vi "CSM-LogViewer(WhileLoop).vi"() -> ()   [LabVIEW 2020]
uses:
  <userlib>/_NEVSTOP/Communicable State Machine(CSM)/_Support/Common/Trim Single line Text.vi
  <userlib>/_NEVSTOP/Communicable State Machine(CSM)/_Support/Common/Format Timestamp.vi
  <userlib>/_NEVSTOP/Communicable State Machine(CSM)/Communicable State Machine.lvlib
panel:
  in  "read line":bool
  in  "stop":bool
  in  "Array":cluster{"CSM":string, "Message":string}[](array[cluster])=[{"CSM"="DH1766", "Message"="MeasureAllVC(Complete)"}, {"CSM"="DH1766", "Message"="MeasureAllVC"}, {"CSM"="IT6900-2", "Message"="MeasureAllVC"}, {"CSM"="IT6900-2", "Message"="MeasureAllVC(Complete)"}, {"CSM"="电流监控", "Message"="Action: Check Current"}, {"CSM"="电流监控", "Message"="Action: Update Status"}, {"CSM"="电流监控", "Message"="Action: Continous Check"}, {"CSM"="电流监控", "Message"="Action: Continous Check(Complete)"}, {"CSM"="YX10A", "Message"="Action: Send R2 and R4"}, {"CSM"="YX10A", "Message"="Action: Continue Check"}, {"CSM"="YX10A", "Message"="Action: Continue Check(Complete)"}]
  out "String Cache":string="[11:08:49.216] [2024/7/18 12:18:43]  [Module Destroyed] CSM-Script-Window\r\n\r[11:08:49.214] [2024/7/18 12:18:43]  [State Change] CSM-Script-Window | <Remaining States> >> <Empty>\r\n\r[11:08:49.212] [2024/7/18 12:18:43]  [State Change] CSM-Script-Window | Exit\r\n\r[11:08:49.210] [2024/7/18 12:18:43]  [State Change] CSM-Script-Window | Events: Unregister\r\n\r[11:08:49.207] [2024/7/18 12:18:43]  [State Change] CSM-Script-Window | Data: Cleanup\r\n\r[11:08:49.205] [2024/7/18 12:18:43]  [State Change] CSM-Script-Window | Macro: Exit(Complete) <- -SendMsgAPI95F21AFF29B0\r\n\r[11:08:49.203] [2024/7/18 12:18:43]  [State Change] CSM-Script-Window | Macro: Exit <- -SendMsgAPI95F21AFF29B0\r\n\r[11:08:49.200] [2024/7/18 12:17:39]  [State Change] CSM-Script-Window | \r\n\r[11:08:49.199] [2024/7/18 12:17:39]  [State Change] Switch2737 | Close(Complete) <- CSM-Script-Window\r\n\r[11:08:49.196] [2024/7/18 12:17:39]  [State Change] Switch2737 | Close <- CSM-Script-Window\r\n\r[11:08:49.194] [2024/7/18 12:17:39]  [User Log] CMD | Close -@ Switch2737\r\n\r[11:08:49.192] [2024/7/18 12:17:39]  [State Change] NI6349DO | Close(Complete) <- CSM-Script-Window\r\n\r[11:08:49.190] [2024/7/18 12:17:39]  [User Log] NI6349DO | Close >> {reset:TRUE}\r\n\r[11:08:49.188] [2024/7/18 12:17:39]  [State Change] NI6349DO | Close <- CSM-Script-Window\r\n\r[11:08:49.186] [2024/7/18 12:17:39]  [User Log] CMD | Close -@ NI6349DO\r\n\r[11:08:49.184] [2024/7/18 12:17:39]  [State Change] NI6509DO | Close(Complete) <- CSM-Script-Window\r\n\r[11:08:49.182] [2024/7/18 12:17:39]  [User Log] NI6509DO | Close >> {reset:TRUE}\r\n\r[11:08:49.180] [2024/7/18 12:17:39]  [State Change] NI6509DO | Close <- CSM-Script-Window\r\n\r[11:08:49.178] [2024/7/18 12:17:39]  [User Log] CMD | Close -@ NI6509DO\r\n\r[11:08:49.176] [2024/7/18 12:17:39]  [State Change] NI6349AI | Close(Complete) <- CSM-Script-Window\r\n\r[11:08:49.174] [2024/7/18 12:17:39]  [State Change] NI6349AI | Close <- CSM-Script-Window\r\n\r[11:08:49.172] [2024/7/18 12:17:39]  [User Log] CMD | Close -@ NI6349AI\r\n\r[11:08:49.170] [2024/7/18 12:17:39]  [State Change] DL850E | Close(Complete) <- CSM-Script-Window\r\n\r[11:08:49.168] [2024/7/18 12:17:39]  [State Change] DL850E | Close <- CSM-Script-Window\r\n\r[11:08:49.166] [2024/7/18 12:17:39]  [User Log] CMD | Close -@ DL850E\r\n\r[11:08:49.164] [2024/7/18 12:17:39]  [State Change] TargetSim | Close(Complete) <- CSM-Script-Window\r\n\r[11:08:49.161] [2024/7/18 12:17:39]  [State Change] TargetSim | Close <- CSM-Script-Window\r\n\r[11:08:49.159] [2024/7/18 12:17:39]  [User Log] CMD | Close -@ TargetSim\r\n\r[11:08:49.157] [2024/7/18 12:17:39]  [State Change] TM10A | Close(Complete) <- CSM-Script-Window\r\n\r[11:08:49.155] [2024/7/18 12:17:39]  [State Change] TM10A | Close <- CSM-Script-Window\r\n\r[11:08:49.153] [2024/7/18 12:17:39]  [User Log] CMD | Close -@ TM10A\r\n\r[11:08:49.151] [2024/7/18 12:17:39]  [State Change] Safe10A | Close(Complete) <- CSM-Script-Window\r\n\r[11:08:49.149] [2024/7/18 12:17:38]  [State Change] Safe10A | Close <- CSM-Script-Window\r\n\r[11:08:49.147] [2024/7/18 12:17:38]  [User Log] CMD | Close -@ Safe10A\r\n\r[11:08:49.145] [2024/7/18 12:17:38]  [State Change] YX10A | Action: Stop Sending R2 and R4(Complete) <- <end>\r\n\r[11:08:49.143] [2024/7/18 12:17:38]  [State Change] YX10A | Action: Stop Sending R2 and R4 <- <end>\r\n\r[11:08:49.141] [2024/7/18 12:17:38]  [State Change] YX10A | Close(Complete) <- CSM-Script-Window\r\n\r[11:08:49.139] [2024/7/18 12:17:38]  [State Change] YX10A | Close <- CSM-Script-Window\r\n\r[11:08:49.137] [2024/7/18 12:17:38]  [User Log] CMD | Close -@ YX10A\r\n\r[11:08:49.135] [2024/7/18 12:17:38]  [State Change] DH1766 | Close(Complete) <- CSM-Script-Window\r\n\r[11:08:48.357] [2024/7/18 12:17:37]  [State Change] DH1766 | Close <- CSM-Script-Window\r\n\r[11:08:48.355] [2024/7/18 12:17:37]  [User Log] CMD | Close -@ DH1766\r\n\r[11:08:48.353] [2024/7/18 12:17:37]  [State Change] DH1766 | Output(Complete) >> FALSE;2 <- CSM-Script-Window\r\n\r[11:08:48.298] [2024/7/18 12:17:37]  [Error Log] Safe10A | Error: -1073807298 >> [Error: -1073807298]VISA Read in Safe.lvlib:Safe(10A).vi%2D%3E10A - COMCSMs.vi%2D%3E10A - CSMs(Without DCPower).vi%2D%3E10A - CSMs.vi\r\n\r[11:08:48.021] [2024/7/18 12:17:37]  [State Change] DH1766 | Output >> FALSE;2 <- CSM-Script-Window\r\n\r[11:08:48.017] [2024/7/18 12:17:37]  [User Log] CMD | Output >> FALSE;2 -@ DH1766\r\n\r[11:08:48.006] [2024/7/18 12:17:36]  [State Change] IT6900-2 | Close(Complete) <- CSM-Script-Window\r\n\r[11:08:47.996] [2024/7/18 12:17:36]  [State Change] IT6900-2 | Close <- CSM-Script-Window\r\n\r[11:08:47.989] [2024/7/18 12:17:36]  [User Log] CMD | Close -@ IT6900-2\r\n\r[11:08:47.988] [2024/7/18 12:17:36]  [State Change] IT6900-2 | Output(Complete) >> FALSE;0 <- CSM-Script-Window\r\n\r[11:08:47.985] [2024/7/18 12:17:36]  [State Change] IT6900-2 | Output >> FALSE;0 <- CSM-Script-Window\r\n\r[11:08:47.983] [2024/7/18 12:17:36]  [User Log] CMD | Output >> FALSE;0 -@ IT6900-2\r\n\r[11:08:47.982] [2024/7/18 12:17:36]  [State Change] 电流监控 | UI: Front Panel State(Complete) >> Close <- CSM-Script-Window\r\n\r[11:08:47.974] [2024/7/18 12:17:36]  [State Change] 电流监控 | UI: Front Panel State >> Close <- CSM-Script-Window\r\n\r[11:08:47.972] [2024/7/18 12:17:36]  [State Change] 电流监控 | Action: Update Status(Complete) <- <end>\r\n\r[11:08:47.965] [2024/7/18 12:17:36]  [User Log] CMD | UI: Front Panel State >> Close -@ 电流监控\r\n\r[11:08:47.961] [2024/7/18 12:17:36]  [State Change] 电流监控 | Action: Finish Monitoring\r\n\r[11:08:47.957] [2024/7/18 12:17:36]  [State Change] 电流监控 | 停止电流监控(Complete) <- CSM-Script-Window\r\n\r[11:08:47.955] [2024/7/18 12:17:36]  [State Change] 电流监控 | 停止电流监控 <- CSM-Script-Window\r\n\r[11:08:47.922] [2024/7/18 12:17:36]  [User Log] CMD | 停止电流监控 -@ 电流监控\r\n\r[11:08:47.908] [2024/7/18 12:17:36]  [State Change] DUTCTRL | ALOG_R(Complete) >> FALSE <- CSM-Script-Window\r\n\r[11:08:47.906] [2024/7/18 12:17:36]  [State Change] NI6509DO | WriteLine(Complete) >> {Line:PXIe-6509/port1/line1;Value:FALSE} <- -SendMsgAPIBD11725CA234\r\n\r[11:08:47.903] [2024/7/18 12:17:36]  [State Change] NI6509DO | WriteLine >> {Line:PXIe-6509/port1/line1;Value:FALSE} <- -SendMsgAPIBD11725CA234\r\n\r[11:08:47.894] [2024/7/18 12:17:36]  [State Change] DUTCTRL | ALOG_R >> FALSE <- CSM-Script-Window\r\n\r[11:08:47.893] [2024/7/18 12:17:36]  [User Log] CMD | ALOG_R >> FALSE -@ DUTCTRL\r\n\r[11:08:47.878] [2024/7/18 12:17:36]  [State Change] DUTCTRL | ALOG(Complete) >> FALSE <- CSM-Script-Window\r\n\r[11:08:47.873] [2024/7/18 12:17:36]  [State Change] NI6349DO | WriteLine(Complete) >> {Line:PXIe-6349/port0/line1;Value:FALSE} <- -SendMsgAPIC0BB74C057F0\r\n\r[11:08:47.867] [2024/7/18 12:17:36]  [State Change] NI6349DO | WriteLine >> {Line:PXIe-6349/port0/line1;Value:FALSE} <- -SendMsgAPIC0BB74C057F0\r\n\r[11:08:47.863] [2024/7/18 12:17:36]  [State Change] DUTCTRL | ALOG >> FALSE <- CSM-Script-Window\r\n\r[11:08:47.861] [2024/7/18 12:17:36]  [User Log] CMD | ALOG >> FALSE -@ DUTCTRL\r\n\r[11:08:47.847] [2024/7/18 12:17:36]  [State Change] DUTCTRL | ES(Complete) >> FALSE <- CSM-Script-Window\r\n\r[11:08:47.845] [2024/7/18 12:17:36]  [State Change] NI6349DO | WriteLine(Complete) >> {Line:PXIe-6349/port0/line0;Value:FALSE} <- -SendMsgAPI295239AE27F2\r\n\r[11:08:47.843] [2024/7/18 12:17:36]  [State Change] NI6349DO | WriteLine >> {Line:PXIe-6349/port0/line0;Value:FALSE} <- -SendMsgAPI295239AE27F2\r\n\r[11:08:47.834] [2024/7/18 12:17:36]  [State Change] DUTCTRL | ES >> FALSE <- CSM-Script-Window\r\n\r[11:08:47.832] [2024/7/18 12:17:36]  [User Log] CMD | ES >> FALSE -@ DUTCTRL\r\n\r[11:08:47.831] [2024/7/18 12:17:36]  [State Change] Switch2737 | DisconnectAll(Complete) <- CSM-Script-Window\r\n\r[11:08:47.829] [2024/7/18 12:17:36]  [State Change] Switch2737 | DisconnectAll <- CSM-Script-Window\r\n\r[11:08:47.827] [2024/7/18 12:17:36]  [User Log] CMD | DisconnectAll -@ Switch2737\r\n\r[11:08:47.825] [2024/7/18 12:17:36]  [State Change] CSM-Script-Window | API: Run Scripts\r\n\r[11:08:47.297] [2024/7/18 12:17:36]  [State Change] CSM-Script-Window | \r\n\r[11:08:47.290] [2024/7/18 12:17:36]  [State Change] CSM-Script-Window | UI: Switch Script\r\n\r[11:08:43.125] [2024/7/18 12:17:29]  [Status] 电压测量 | Operation Log >> 测量电压: FZ_Laser 值为35.485611\r\n\r[11:08:43.122] [2024/7/18 12:17:29]  [Status] 电压测量 | Report Data >> <MassData>Start:625190;Size:51\r\n\r[11:08:43.120] [2024/7/18 12:17:29]  [Status] 电压测量 | Operation Log >> FZ_Laser: 35.485611\r\n\r[11:08:43.118] [2024/7/18 12:17:29]  [State Change] 电压测量 | 测量电压(Complete) >> FZ_Laser <- Tool-Testpnl\r\n\r[11:08:42.497] [2024/7/18 12:17:28]  [State Change] NI6349AI | ReadN(Complete) >> 24;200 <- -SendMsgAPI649D389687CA\r\n\r[11:08:42.174] [2024/7/18 12:17:28]  [State Change] NI6349AI | ReadN >> 24;200 <- -SendMsgAPI649D389687CA\r\n\r[11:08:42.172] [2024/7/18 12:17:28]  [State Change] 电压测量 | 测量电压 >> FZ_Laser <- Tool-Testpnl\r\n\r[11:08:41.196] [2024/7/18 12:17:26]  [Status] 电压测量 | Operation Log >> 测量电压: FZ_Laser 值为35.428351\r\n\r[11:08:41.194] [2024/7/18 12:17:26]  [Status] 电压测量 | Report Data >> <MassData>Start:495495;Size:51\r\n\r[11:08:41.192] [2024/7/18 12:17:26]  [Status] 电压测量 | Operation Log >> FZ_Laser: 35.428351\r\n\r[11:08:41.190] [2024/7/18 12:17:26]  [State Change] 电压测量 | 测量电压(Complete) >> FZ_Laser <- Tool-Testpnl\r\n\r[11:08:40.530] [2024/7/18 12:17:25]  [State Change] NI6349AI | ReadN(Complete) >> 24;200 <- -SendMsgAPI649D389687CA\r\n\r[11:08:40.210] [2024/7/18 12:17:25]  [State Change] NI6349AI | ReadN >> 24;200 <- -SendMsgAPI649D389687CA\r\n\r[11:08:40.208] [2024/7/18 12:17:25]  [State Change] 电压测量 | 测量电压 >> FZ_Laser <- Tool-Testpnl\r\n\r[11:08:39.289] [2024/7/18 12:17:24]  [Status] 电压测量 | Operation Log >> 测量电压: FZ_Laser 值为35.553098\r\n\r[11:08:39.287] [2024/7/18 12:17:24]  [Status] 电压测量 | Report Data >> <MassData>Start:365800;Size:51\r\n\r[11:08:39.285] [2024/7/18 12:17:24]  [Status] 电压测量 | Operation Log >> FZ_Laser: 35.553098\r\n\r[11:08:39.283] [2024/7/18 12:17:24]  [State Change] 电压测量 | 测量电压(Complete) >> FZ_Laser <- Tool-Testpnl\r\n\r[11:08:38.289] [2024/7/18 12:17:22]  [State Ch"
  out "XY Graph":T1(graph)=[{timestamp(3804120837 s since 1904-01-01), "offset (in bytes) (0)"=19}, {timestamp(3804120838 s since 1904-01-01), "offset (in bytes) (0)"=21}, {timestamp(3804120839 s since 1904-01-01), "offset (in bytes) (0)"=16}, {timestamp(3804120840 s since 1904-01-01), "offset (in bytes) (0)"=19}, {timestamp(3804120841 s since 1904-01-01), "offset (in bytes) (0)"=18}, {timestamp(3804120842 s since 1904-01-01), "offset (in bytes) (0)"=19}, {timestamp(3804120843 s since 1904-01-01), "offset (in bytes) (0)"=24}, {timestamp(3804120844 s since 1904-01-01), "offset (in bytes) (0)"=24}, {timestamp(3804120845 s since 1904-01-01), "offset (in bytes) (0)"=19}, {timestamp(3804120846 s since 1904-01-01), "offset (in bytes) (0)"=55}, {timestamp(3804120847 s since 1904-01-01), "offset (in bytes) (0)"=1}, {timestamp(3804120851 s since 1904-01-01), "offset (in bytes) (0)"=10}, {timestamp(3804120852 s since 1904-01-01), "offset (in bytes) (0)"=35}, {timestamp(3804120853 s since 1904-01-01), "offset (in bytes) (0)"=16}, {timestamp(3804120854 s since 1904-01-01), "offset (in bytes) (0)"=19}, {timestamp(3804120855 s since 1904-01-01), "offset (in bytes) (0)"=21}, {timestamp(3804120856 s since 1904-01-01), "offset (in bytes) (0)"=16}, {timestamp(3804120857 s since 1904-01-01), "offset (in bytes) (0)"=19}, {timestamp(3804120858 s since 1904-01-01), "offset (in bytes) (0)"=21}, {timestamp(3804120859 s since 1904-01-01), "offset (in bytes) (0)"=16}, {timestamp(3804120860 s since 1904-01-01), "offset (in bytes) (0)"=19}, {timestamp(3804120861 s since 1904-01-01), "offset (in bytes) (0)"=18}, {timestamp(3804120862 s since 1904-01-01), "offset (in bytes) (0)"=19}, {timestamp(3804120863 s since 1904-01-01), "offset (in bytes) (0)"=19}, {timestamp(3804120864 s since 1904-01-01), "offset (in bytes) (0)"=26}, {timestamp(3804120865 s since 1904-01-01), "offset (in bytes) (0)"=20}, {timestamp(3804120866 s since 1904-01-01), "offset (in bytes) (0)"=19}, {timestamp(3804120867 s since 1904-01-01), "offset (in bytes) (0)"=16}, {timestamp(3804120868 s since 1904-01-01), "offset (in bytes) (0)"=21}, {timestamp(3804120869 s since 1904-01-01), "offset (in bytes) (0)"=19}, {timestamp(3804120870 s since 1904-01-01), "offset (in bytes) (0)"=25}, {timestamp(3804120871 s since 1904-01-01), "offset (in bytes) (0)"=29}, {timestamp(3804120872 s since 1904-01-01), "offset (in bytes) (0)"=20}, {timestamp(3804120873 s since 1904-01-01), "offset (in bytes) (0)"=16}, {timestamp(3804120874 s since 1904-01-01), "offset (in bytes) (0)"=30}, {timestamp(3804120875 s since 1904-01-01), "offset (in bytes) (0)"=26}, {timestamp(3804120876 s since 1904-01-01), "offset (in bytes) (0)"=45}, {timestamp(3804120877 s since 1904-01-01), "offset (in bytes) (0)"=37}, {timestamp(3804120878 s since 1904-01-01), "offset (in bytes) (0)"=39}, {timestamp(3804120879 s since 1904-01-01), "offset (in bytes) (0)"=23}, {timestamp(3804120880 s since 1904-01-01), "offset (in bytes) (0)"=36}, {timestamp(3804120881 s since 1904-01-01), "offset (in bytes) (0)"=21}, {timestamp(3804120882 s since 1904-01-01), "offset (in bytes) (0)"=26}, {timestamp(3804120883 s since 1904-01-01), "offset (in bytes) (0)"=21}, {timestamp(3804120884 s since 1904-01-01), "offset (in bytes) (0)"=31}, {timestamp(3804120885 s since 1904-01-01), "offset (in bytes) (0)"=21}, {timestamp(3804120886 s since 1904-01-01), "offset (in bytes) (0)"=23}, {timestamp(3804120887 s since 1904-01-01), "offset (in bytes) (0)"=28}, {timestamp(3804120888 s since 1904-01-01), "offset (in bytes) (0)"=27}, {timestamp(3804120889 s since 1904-01-01), "offset (in bytes) (0)"=27}, {timestamp(3804120890 s since 1904-01-01), "offset (in bytes) (0)"=19}, {timestamp(3804120891 s since 1904-01-01), "offset (in bytes) (0)"=34}, {timestamp(3804120892 s since 1904-01-01), "offset (in bytes) (0)"=20}, {timestamp(3804120893 s since 1904-01-01), "offset (in bytes) (0)"=23}, {timestamp(3804120894 s since 1904-01-01), "offset (in bytes) (0)"=29}, {timestamp(3804120895 s since 1904-01-01), "offset (in bytes) (0)"=26}, {timestamp(3804120896 s since 1904-01-01), "offset (in bytes) (0)"=28}, {timestamp(3804120897 s since 1904-01-01), "offset (in bytes) (0)"=19}, {timestamp(3804120898 s since 1904-01-01), "offset (in bytes) (0)"=22}, {timestamp(3804120899 s since 1904-01-01), "offset (in bytes) (0)"=32}, {timestamp(3804120900 s since 1904-01-01), "offset (in bytes) (0)"=19}, {timestamp(3804120901 s since 1904-01-01), "offset (in bytes) (0)"=28}, {timestamp(3804120902 s since 1904-01-01), "offset (in bytes) (0)"=30}, {timestamp(3804120903 s since 1904-01-01), "offset (in bytes) (0)"=29}, {timestamp(3804120904 s since 1904-01-01), "offset (in bytes) (0)"=16}, {timestamp(3804120905 s since 1904-01-01), "offset (in bytes) (0)"=25}, {timestamp(3804120906 s since 1904-01-01), "offset (in bytes) (0)"=32}, {timestamp(3804120907 s since 1904-01-01), "offset (in bytes) (0)"=16}, {timestamp(3804120908 s since 1904-01-01), "offset (in bytes) (0)"=25}, {timestamp(3804120909 s since 1904-01-01), "offset (in bytes) (0)"=38}, {timestamp(3804120910 s since 1904-01-01), "offset (in bytes) (0)"=18}, {timestamp(3804120911 s since 1904-01-01), "offset (in bytes) (0)"=25}, {timestamp(3804120912 s since 1904-01-01), "offset (in bytes) (0)"=32}, {timestamp(3804120913 s since 1904-01-01), "offset (in bytes) (0)"=18}, {timestamp(3804120914 s since 1904-01-01), "offset (in bytes) (0)"=39}, {timestamp(3804120915 s since 1904-01-01), "offset (in bytes) (0)"=19}, {timestamp(3804120916 s since 1904-01-01), "offset (in bytes) (0)"=29}, {timestamp(3804120917 s since 1904-01-01), "offset (in bytes) (0)"=22}, {timestamp(3804120918 s since 1904-01-01), "offset (in bytes) (0)"=19}, {timestamp(3804120919 s since 1904-01-01), "offset (in bytes) (0)"=25}, {timestamp(3804120920 s since 1904-01-01), "offset (in bytes) (0)"=29}, {timestamp(3804120921 s since 1904-01-01), "offset (in bytes) (0)"=20}, {timestamp(3804120922 s since 1904-01-01), "offset (in bytes) (0)"=50}, {timestamp(3804120923 s since 1904-01-01), "offset (in bytes) (0)"=308}, {timestamp(3804120924 s since 1904-01-01), "offset (in bytes) (0)"=327}, {timestamp(3804120925 s since 1904-01-01), "offset (in bytes) (0)"=317}, {timestamp(3804120926 s since 1904-01-01), "offset (in bytes) (0)"=330}, {timestamp(3804120927 s since 1904-01-01), "offset (in bytes) (0)"=336}, {timestamp(3804120928 s since 1904-01-01), "offset (in bytes) (0)"=316}, {timestamp(3804120929 s since 1904-01-01), "offset (in bytes) (0)"=323}, {timestamp(3804120930 s since 1904-01-01), "offset (in bytes) (0)"=323}, {timestamp(3804120931 s since 1904-01-01), "offset (in bytes) (0)"=320}, {timestamp(3804120932 s since 1904-01-01), "offset (in bytes) (0)"=327}, {timestamp(3804120933 s since 1904-01-01), "offset (in bytes) (0)"=327}, {timestamp(3804120934 s since 1904-01-01), "offset (in bytes) (0)"=316}, {timestamp(3804120935 s since 1904-01-01), "offset (in bytes) (0)"=330}, {timestamp(3804120936 s since 1904-01-01), "offset (in bytes) (0)"=317}, {timestamp(3804120937 s since 1904-01-01), "offset (in bytes) (0)"=319}, {timestamp(3804120938 s since 1904-01-01), "offset (in bytes) (0)"=321}, {timestamp(3804120939 s since 1904-01-01), "offset (in bytes) (0)"=316}, {timestamp(3804120940 s since 1904-01-01), "offset (in bytes) (0)"=319}, {timestamp(3804120941 s since 1904-01-01), "offset (in bytes) (0)"=321}, {timestamp(3804120942 s since 1904-01-01), "offset (in bytes) (0)"=316}, {timestamp(3804120943 s since 1904-01-01), "offset (in bytes) (0)"=319}, {timestamp(3804120944 s since 1904-01-01), "offset (in bytes) (0)"=321}, {timestamp(3804120945 s since 1904-01-01), "offset (in bytes) (0)"=316}, {timestamp(3804120946 s since 1904-01-01), "offset (in bytes) (0)"=319}, {timestamp(3804120947 s since 1904-01-01), "offset (in bytes) (0)"=321}, {timestamp(3804120948 s since 1904-01-01), "offset (in bytes) (0)"=316}, {timestamp(3804120949 s since 1904-01-01), "offset (in bytes) (0)"=319}, {timestamp(3804120950 s since 1904-01-01), "offset (in bytes) (0)"=321}, {timestamp(3804120951 s since 1904-01-01), "offset (in bytes) (0)"=316}, {timestamp(3804120952 s since 1904-01-01), "offset (in bytes) (0)"=319}, {timestamp(3804120953 s since 1904-01-01), "offset (in bytes) (0)"=321}, {timestamp(3804120954 s since 1904-01-01), "offset (in bytes) (0)"=316}, {timestamp(3804120955 s since 1904-01-01), "offset (in bytes) (0)"=319}, {timestamp(3804120956 s since 1904-01-01), "offset (in bytes) (0)"=321}, {timestamp(3804120957 s since 1904-01-01), "offset (in bytes) (0)"=316}, {timestamp(3804120958 s since 1904-01-01), "offset (in bytes) (0)"=319}, {timestamp(3804120959 s since 1904-01-01), "offset (in bytes) (0)"=321}, {timestamp(3804120960 s since 1904-01-01), "offset (in bytes) (0)"=313}, {timestamp(3804120961 s since 1904-01-01), "offset (in bytes) (0)"=319}, {timestamp(3804120962 s since 1904-01-01), "offset (in bytes) (0)"=321}, {timestamp(3804120963 s since 1904-01-01), "offset (in bytes) (0)"=316}, {timestamp(3804120964 s since 1904-01-01), "offset (in bytes) (0)"=319}, {timestamp(3804120965 s since 1904-01-01), "offset (in bytes) (0)"=321}, {timestamp(3804120966 s since 1904-01-01), "offset (in bytes) (0)"=316}, {timestamp(3804120967 s since 1904-01-01), "offset (in bytes) (0)"=319}, {timestamp(3804120968 s since 1904-01-01), "offset (in bytes) (0)"=321}, {timestamp(3804120969 s since 1904-01-01), "offset (in bytes) (0)"=316}, {timestamp(3804120970 s since 1904-01-01), "offset (in bytes) (0)"=321}, {timestamp(3804120971 s since 1904-01-01), "offset (in bytes) (0)"=321}, {timestamp(3804120972 s since 1904-01-01), "offset (in bytes) (0)"=316}, {timestamp(3804120973 s since 1904-01-01), "offset (in bytes) (0)"=319}, {timestamp(3804120974 s since 1904-01-01), "offset (in bytes) (0)"=321}, {timestamp(3804120975 s since 1904-01-01), "offset (in bytes) (0)"=316}, {timestamp(3804120976 s since 1904-01-01), "offset (in bytes) (0)"=319}, {timestamp(3804120977 s since 1904-01-01), "offset (in bytes) (0)"=322}, {timestamp(3804120978 s since 1904-01-01), "offset (in bytes) (0)"=317}, {timestamp(3804120979 s since 1904-01-01), "offset (in bytes) (0)"=319}, {timestamp(3804120980 s since 1904-01-01), "offset (in bytes) (0)"=320}, {timestamp(3804120981 s since 1904-01-01), "offset (in bytes) (0)"=319}, {timestamp(3804120982 s since 1904-01-01), "offset (in bytes) (0)"=319}, {timestamp(3804120983 s since 1904-01-01), "offset (in bytes) (0)"=318}, {timestamp(3804120984 s since 1904-01-01), "offset (in bytes) (0)"=319}, {timestamp(3804120985 s since 1904-01-01), "offset (in bytes) (0)"=319}, {timestamp(3804120986 s since 1904-01-01), "offset (in bytes) (0)"=318}, {timestamp(3804120987 s since 1904-01-01), "offset (in bytes) (0)"=319}, {timestamp(3804120988 s since 1904-01-01), "offset (in bytes) (0)"=319}, {timestamp(3804120989 s since 1904-01-01), "offset (in bytes) (0)"=318}, {timestamp(3804120990 s since 1904-01-01), "offset (in bytes) (0)"=319}, {timestamp(3804120991 s since 1904-01-01), "offset (in bytes) (0)"=319}, {timestamp(3804120992 s since 1904-01-01), "offset (in bytes) (0)"=318}, {timestamp(3804120993 s since 1904-01-01), "offset (in bytes) (0)"=319}, {timestamp(3804120994 s since 1904-01-01), "offset (in bytes) (0)"=319}, {timestamp(3804120995 s since 1904-01-01), "offset (in bytes) (0)"=316}, {timestamp(3804120996 s since 1904-01-01), "offset (in bytes) (0)"=321}, {timestamp(3804120997 s since 1904-01-01), "offset (in bytes) (0)"=321}, {timestamp(3804120998 s since 1904-01-01), "offset (in bytes) (0)"=316}, {timestamp(3804120999 s since 1904-01-01), "offset (in bytes) (0)"=321}, {timestamp(3804121000 s since 1904-01-01), "offset (in bytes) (0)"=319}, {timestamp(3804121001 s since 1904-01-01), "offset (in bytes) (0)"=316}, {timestamp(3804121002 s since 1904-01-01), "offset (in bytes) (0)"=321}, {timestamp(3804121003 s since 1904-01-01), "offset (in bytes) (0)"=321}, {timestamp(3804121004 s since 1904-01-01), "offset (in bytes) (0)"=316}, {timestamp(3804121005 s since 1904-01-01), "offset (in bytes) (0)"=321}, {timestamp(3804121006 s since 1904-01-01), "offset (in bytes) (0)"=319}, {timestamp(3804121007 s since 1904-01-01), "offset (in bytes) (0)"=316}, {timestamp(3804121008 s since 1904-01-01), "offset (in bytes) (0)"=321}, {timestamp(3804121009 s since 1904-01-01), "offset (in bytes) (0)"=321}, {timestamp(3804121010 s since 1904-01-01), "offset (in bytes) (0)"=317}, {timestamp(3804121011 s since 1904-01-01), "offset (in bytes) (0)"=325}, {timestamp(3804121012 s since 1904-01-01), "offset (in bytes) (0)"=319}, {timestamp(3804121013 s since 1904-01-01), "offset (in bytes) (0)"=318}, {timestamp(3804121014 s since 1904-01-01), "offset (in bytes) (0)"=322}, {timestamp(3804121015 s since 1904-01-01), "offset (in bytes) (0)"=323}, {timestamp(3804121016 s since 1904-01-01), "offset (in bytes) (0)"=318}, {timestamp(3804121017 s since 1904-01-01), "offset (in bytes) (0)"=323}, {timestamp(3804121018 s since 1904-01-01), "offset (in bytes) (0)"=319}, {timestamp(3804121019 s since 1904-01-01), "offset (in bytes) (0)"=319}, {timestamp(3804121020 s since 1904-01-01), "offset (in bytes) (0)"=321}, {timestamp(3804121021 s since 1904-01-01), "offset (in bytes) (0)"=319}, {timestamp(3804121022 s since 1904-01-01), "offset (in bytes) (0)"=316}, {timestamp(3804121023 s since 1904-01-01), "offset (in bytes) (0)"=321}, {timestamp(3804121024 s since 1904-01-01), "offset (in bytes) (0)"=319}, {timestamp(3804121025 s since 1904-01-01), "offset (in bytes) (0)"=316}, {timestamp(3804121026 s since 1904-01-01), "offset (in bytes) (0)"=321}, {timestamp(3804121027 s since 1904-01-01), "offset (in bytes) (0)"=323}, {timestamp(3804121028 s since 1904-01-01), "offset (in bytes) (0)"=316}, {timestamp(3804121029 s since 1904-01-01), "offset (in bytes) (0)"=321}, {timestamp(3804121030 s since 1904-01-01), "offset (in bytes) (0)"=319}, {timestamp(3804121031 s since 1904-01-01), "offset (in bytes) (0)"=318}, {timestamp(3804121032 s since 1904-01-01), "offset (in bytes) (0)"=322}, {timestamp(3804121033 s since 1904-01-01), "offset (in bytes) (0)"=323}, {timestamp(3804121034 s since 1904-01-01), "offset (in bytes) (0)"=316}, {timestamp(3804121035 s since 1904-01-01), "offset (in bytes) (0)"=312}, {timestamp(3804121036 s since 1904-01-01), "offset (in bytes) (0)"=319}, {timestamp(3804121037 s since 1904-01-01), "offset (in bytes) (0)"=316}, {timestamp(3804121038 s since 1904-01-01), "offset (in bytes) (0)"=321}, {timestamp(3804121039 s since 1904-01-01), "offset (in bytes) (0)"=310}, {timestamp(3804121040 s since 1904-01-01), "offset (in bytes) (0)"=319}, {timestamp(3804121041 s since 1904-01-01), "offset (in bytes) (0)"=323}, {timestamp(3804121042 s since 1904-01-01), "offset (in bytes) (0)"=317}, {timestamp(3804121043 s since 1904-01-01), "offset (in bytes) (0)"=319}, {timestamp(3804121044 s since 1904-01-01), "offset (in bytes) (0)"=325}, {timestamp(3804121045 s since 1904-01-01), "offset (in bytes) (0)"=319}, {timestamp(3804121046 s since 1904-01-01), "offset (in bytes) (0)"=323}, {timestamp(3804121047 s since 1904-01-01), "offset (in bytes) (0)"=318}, {timestamp(3804121048 s since 1904-01-01), "offset (in bytes) (0)"=319}, {timestamp(3804121049 s since 1904-01-01), "offset (in bytes) (0)"=323}, {timestamp(3804121050 s since 1904-01-01), "offset (in bytes) (0)"=321}, {timestamp(3804121051 s since 1904-01-01), "offset (in bytes) (0)"=316}, {timestamp(3804121052 s since 1904-01-01), "offset (in bytes) (0)"=319}, {timestamp(3804121053 s since 1904-01-01), "offset (in bytes) (0)"=321}, {timestamp(3804121054 s since 1904-01-01), "offset (in bytes) (0)"=316}, {timestamp(3804121055 s since 1904-01-01), "offset (in bytes) (0)"=319}, {timestamp(3804121056 s since 1904-01-01), "offset (in bytes) (0)"=355}, {timestamp(3804121057 s since 1904-01-01), "offset (in bytes) (0)"=303}, {timestamp(3804121058 s since 1904-01-01), "offset (in bytes) (0)"=194}, {timestamp(3804121059 s since 1904-01-01), "offset (in bytes) (0)"=25}, {timestamp(3804121123 s since 1904-01-01), "offset (in bytes) (0)"=7}]
  in  "Tree":string(tree)="CMD/采集波形数据"
  out "Variant":variant=variant("CMD | ALOG"=variant(i64 2), "CMD | ALOG_R"=variant(i64 2), "CMD | Close"=variant(i64 11), "CMD | DisconnectAll"=variant(i64 6), "CMD | ES"=variant(i64 2), "CMD | FUSE_R1"=variant(i64 5), "CMD | FUSE_R3"=variant(i64 2), "CMD | Output"=variant(i64 3), "CMD | SafeOutput"=variant(i64 1), "CMD | UI: Front Panel State"=variant(i64 1), "CMD | Wait"=variant(i64 7), "CMD | 采集波形数据"=variant(i64 1), "CMD | 测量电流"=variant(i64 3), "CMD | 测量电压"=variant(i64 14), "CMD | 测量频率"=variant(i64 9), "CMD | 发送自检指令"=variant(i64 1), "CMD | 开始模拟安保返回信息"=variant(i64 1), "CMD | 开始周期发送R2+R4"=variant(i64 1), "CMD | 模拟有目标"=variant(i64 5), "CMD | 全关"=variant(i64 6), "CMD | 设置参数"=variant(i64 5), "CMD | 停止电流监控"=variant(i64 1), "CMD | 延时启动信号"=variant(i64 1), "CMD | 自检时间"=variant(i64 1), "CSM-Script-Window\r\n"=variant(i64 1), "CSM-Script-Window | \r\n"=variant(i64 6), "CSM-Script-Window | <Remaining States>"=variant(i64 1), "CSM-Script-Window | API: Run Scripts\r\n"=variant(i64 2), "CSM-Script-Window | Data: Cleanup\r\n"=variant(i64 1), "CSM-Script-Window | Events: Unregister\r\n"=variant(i64 1), "CSM-Script-Window | Exit\r\n"=variant(i64 1), "CSM-Script-Window | Macro: Exit"=variant(i64 1), "CSM-Script-Window | Macro: Exit(Complete)"=variant(i64 1), "CSM-Script-Window | UI: Switch Script\r\n"=variant(i64 4), "DH1766 | Close"=variant(i64 1), "DH1766 | Close(Complete)"=variant(i64 1), "DH1766 | Data: Get Internal Data"=variant(i64 1), "DH1766 | Data: Get Internal Data(Complete)"=variant(i64 1), "DH1766 | MeasureAll"=variant(i64 1), "DH1766 | MeasureAll(Complete)"=variant(i64 1), "DH1766 | MeasureAllVC"=variant(i64 501), "DH1766 | MeasureAllVC(Complete)"=variant(i64 501), "DH1766 | Output"=variant(i64 2), "DH1766 | Output(Complete)"=variant(i64 2), "DL850E | Acquire"=variant(i64 1), "DL850E | Acquire(Complete)"=variant(i64 1), "DL850E | Close"=variant(i64 1), "DL850E | Close(Complete)"=variant(i64 1), "DL850E | ConfigureAutoTrigger"=variant(i64 12), "DL850E | ConfigureAutoTrigger(Complete)"=variant(i64 12), "DL850E | ConfigureTimeBase"=variant(i64 1), "DL850E | ConfigureTimeBase(Complete)"=variant(i64 1), "DL850E | ConfigureTimebase"=variant(i64 12), "DL850E | ConfigureTimebase(Complete)"=variant(i64 12), "DL850E | ConfigureTrigger"=variant(i64 1), "DL850E | ConfigureTrigger(Complete)"=variant(i64 1), "DL850E | ConfigureVertical"=variant(i64 14), "DL850E | ConfigureVertical(Complete)"=variant(i64 14), "DL850E | Measure"=variant(i64 12), "DL850E | Measure(Complete)"=variant(i64 12), "DUTCTRL | ALOG"=variant(i64 2), "DUTCTRL | ALOG(Complete)"=variant(i64 2), "DUTCTRL | ALOG_R"=variant(i64 2), "DUTCTRL | ALOG_R(Complete)"=variant(i64 2), "DUTCTRL | ES"=variant(i64 2), "DUTCTRL | ES(Complete)"=variant(i64 2), "DUTCTRL | Wait"=variant(i64 7), "DUTCTRL | Wait(Complete)"=variant(i64 7), "IT6900-2 | Close"=variant(i64 1), "IT6900-2 | Close(Complete)"=variant(i64 1), "IT6900-2 | MeasureAll"=variant(i64 2), "IT6900-2 | MeasureAll(Complete)"=variant(i64 2), "IT6900-2 | MeasureAllVC"=variant(i64 501), "IT6900-2 | MeasureAllVC(Complete)"=variant(i64 501), "IT6900-2 | Output"=variant(i64 1), "IT6900-2 | Output(Complete)"=variant(i64 1), "IT6900-2 | SafeOutput"=variant(i64 1), "IT6900-2 | SafeOutput(Complete)"=variant(i64 1), "NI6349AI | Close"=variant(i64 1), "NI6349AI | Close(Complete)"=variant(i64 1), "NI6349AI | ReadN"=variant(i64 19), "NI6349AI | ReadN(Complete)"=variant(i64 19), "NI6349DO | Close"=variant(i64 2), "NI6349DO | Close(Complete)"=variant(i64 1), "NI6349DO | WriteLine"=variant(i64 4), "NI6349DO | WriteLine(Complete)"=variant(i64 4), "NI6509DO | Close"=variant(i64 2), "NI6509DO | Close(Complete)"=variant(i64 1), "NI6509DO | WriteLine"=variant(i64 2), "NI6509DO | WriteLine(Complete)"=variant(i64 2), "Result | +27V电流"=variant(i64 2), "Result | +5V电流"=variant(i64 1), "Result | FZ_Laser"=variant(i64 1), "Result | FZ_UC"=variant(i64 2), "Result | FZ_UP"=variant(i64 1), "Result | FZ_VA_T"=variant(i64 4), "Result | FZ_VB_T"=variant(i64 4), "Result | NOISEA"=variant(i64 1), "Result | NOISEB"=variant(i64 1), "Result | V+12V"=variant(i64 1), "Result | V+15V"=variant(i64 1), "Result | V+5V"=variant(i64 1), "Result | V-5V"=variant(i64 1), "Result | VCLOCK1"=variant(i64 1), "Result | V_+27_CF"=variant(i64 2), "Result | V_ALOG_H"=variant(i64 2), "Result | 发送自检指令"=variant(i64 1), "Result | 自检时间"=variant(i64 1), "Safe10A | Close"=variant(i64 1), "Safe10A | Close(Complete)"=variant(i64 1), "Safe10A | Error: -1073807298"=variant(i64 1), "Safe10A | 工作模式自炸\r\n"=variant(i64 1), "Safe10A | 开始模拟安保返回信息"=variant(i64 1), "Safe10A | 开始模拟安保返回信息(Complete)"=variant(i64 1), "SafeCOM | Read:"=variant(i64 3), "SafeCOM | WRITE:"=variant(i64 1), "Switch2737 | Close"=variant(i64 1), "Switch2737 | Close(Complete)"=variant(i64 1), "Switch2737 | Connect"=variant(i64 14), "Switch2737 | Connect(Complete)"=variant(i64 14), "Switch2737 | DisconnectAll"=variant(i64 6), "Switch2737 | DisconnectAll(Complete)"=variant(i64 6), "TM10A | Close"=variant(i64 1), "TM10A | Close(Complete)"=variant(i64 1), "TargetSim | COM发送"=variant(i64 16), "TargetSim | COM接收"=variant(i64 16), "TargetSim | Close"=variant(i64 1), "TargetSim | Close(Complete)"=variant(i64 1), "TargetSim | 模拟有目标"=variant(i64 5), "TargetSim | 模拟有目标(Complete)"=variant(i64 5), "TargetSim | 模拟有目标A"=variant(i64 5), "TargetSim | 模拟有目标B"=variant(i64 5), "TargetSim | 全关"=variant(i64 6), "TargetSim | 全关(Complete)"=variant(i64 6), "YX10A | Action: Continue Check"=variant(i64 13547), "YX10A | Action: Continue Check(Complete)"=variant(i64 13547), "YX10A | Action: Record SelfTest Start Time\r\n"=variant(i64 1), "YX10A | Action: Record SelfTest Stop Time\r\n"=variant(i64 1), "YX10A | Action: Send R2 and R4\r\n"=variant(i64 13548), "YX10A | Action: Stop Sending R2 and R4"=variant(i64 1), "YX10A | Action: Stop Sending R2 and R4(Complete)"=variant(i64 1), "YX10A | Close"=variant(i64 1), "YX10A | Close(Complete)"=variant(i64 1), "YX10A | FUSE_R1"=variant(i64 5), "YX10A | FUSE_R1\r\n"=variant(i64 1), "YX10A | FUSE_R1(Complete)"=variant(i64 5), "YX10A | FUSE_R3"=variant(i64 2), "YX10A | FUSE_R3(Complete)"=variant(i64 2), "YX10A | FUSE_S1\r\n"=variant(i64 1), "YX10A | 发送自检指令"=variant(i64 1), "YX10A | 发送自检指令(Complete)"=variant(i64 1), "YX10A | 开始周期发送R2+R4"=variant(i64 1), "YX10A | 开始周期发送R2+R4(Complete)"=variant(i64 1), "YX10A | 设置参数"=variant(i64 5), "YX10A | 设置参数(Complete)"=variant(i64 5), "YX10A | 自检时间"=variant(i64 1), "YX10A | 自检时间\r\n"=variant(i64 1), "YX10A | 自检时间(Complete)"=variant(i64 1), "YXCOM | Read:"=variant(i64 3), "YXCOM | WRITE:"=variant(i64 24), "点火及延时信号测试 | API"=variant(i64 1), "点火及延时信号测试 | Error Handler"=variant(i64 1), "点火及延时信号测试 | Error Occurred"=variant(i64 1), "点火及延时信号测试 | Operation Log"=variant(i64 1), "点火及延时信号测试 | Report Data"=variant(i64 1), "点火及延时信号测试 | 采集波形数据"=variant(i64 1), "点火及延时信号测试 | 采集波形数据(Complete)"=variant(i64 1), "点火及延时信号测试 | 延时启动信号"=variant(i64 1), "点火及延时信号测试 | 延时启动信号(Complete)"=variant(i64 1), "电流测量 | Operation Log"=variant(i64 6), "电流测量 | Report Data"=variant(i64 3), "电流测量 | 测量电流"=variant(i64 3), "电流测量 | 测量电流(Complete)"=variant(i64 3), "电流监控 | Action: Check Current\r\n"=variant(i64 501), "电流监控 | Action: Continous Check"=variant(i64 500), "电流监控 | Action: Continous Check(Complete)"=variant(i64 501), "电流监控 | Action: Finish Monitoring\r\n"=variant(i64 1), "电流监控 | Action: Update Status"=variant(i64 1), "电流监控 | Action: Update Status\r\n"=variant(i64 500), "电流监控 | Action: Update Status(Complete)"=variant(i64 1), "电流监控 | UI: Front Panel State"=variant(i64 1), "电流监控 | UI: Front Panel State(Complete)"=variant(i64 1), "电流监控 | 停止电流监控"=variant(i64 1), "电流监控 | 停止电流监控(Complete)"=variant(i64 1), "电压测量 | Data: Get Internal Data"=variant(i64 1), "电压测量 | Data: Get Internal Data(Complete)"=variant(i64 1), "电压测量 | Operation Log"=variant(i64 44), "电压测量 | Report Data"=variant(i64 22), "电压测量 | 测量电压"=variant(i64 22), "电压测量 | 测量电压(Complete)"=variant(i64 22), "频率测量 | Operation Log"=variant(i64 18), "频率测量 | Report Data"=variant(i64 9), "频率测量 | 测量频率"=variant(i64 9), "频率测量 | 测量频率(Complete)"=variant(i64 9))
  out "data":string="[2024/7/18 12:18:43]  [Module Destroyed] CSM-Script-Window"
  out "offset (in bytes) (0)":i64=3621179 format="%.3p"
  out "size":i64=3621239 format="%.3p"
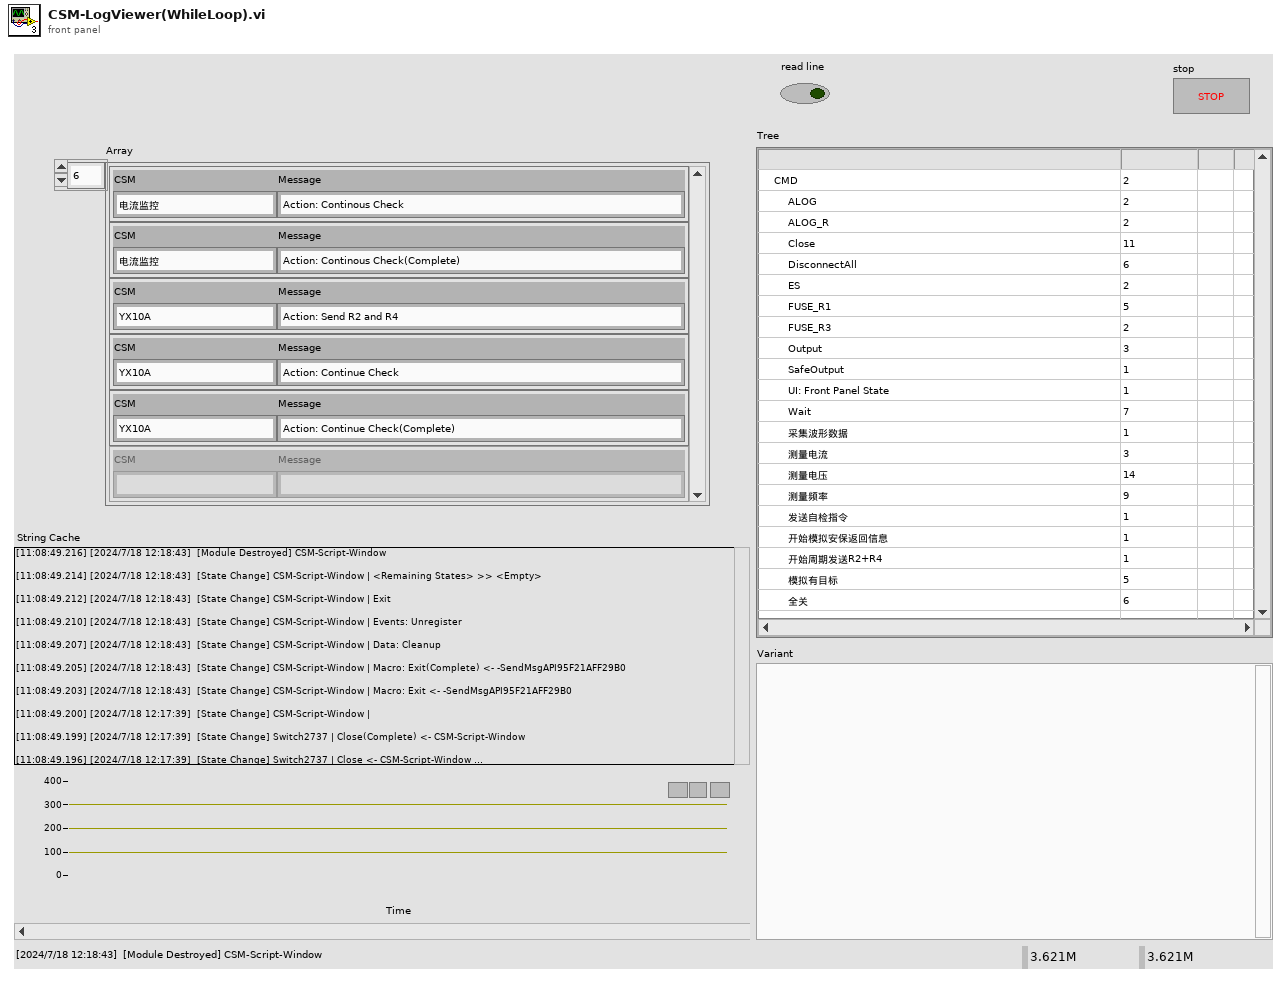
[diagram p1: front panel]
types:
  T1 = cluster{timestamp, "offset (in bytes) (0)":i64}[]
  T2 = enum16{"open", "replace", "create", "open or create", "replace or create", "replace or create with confirmation"}
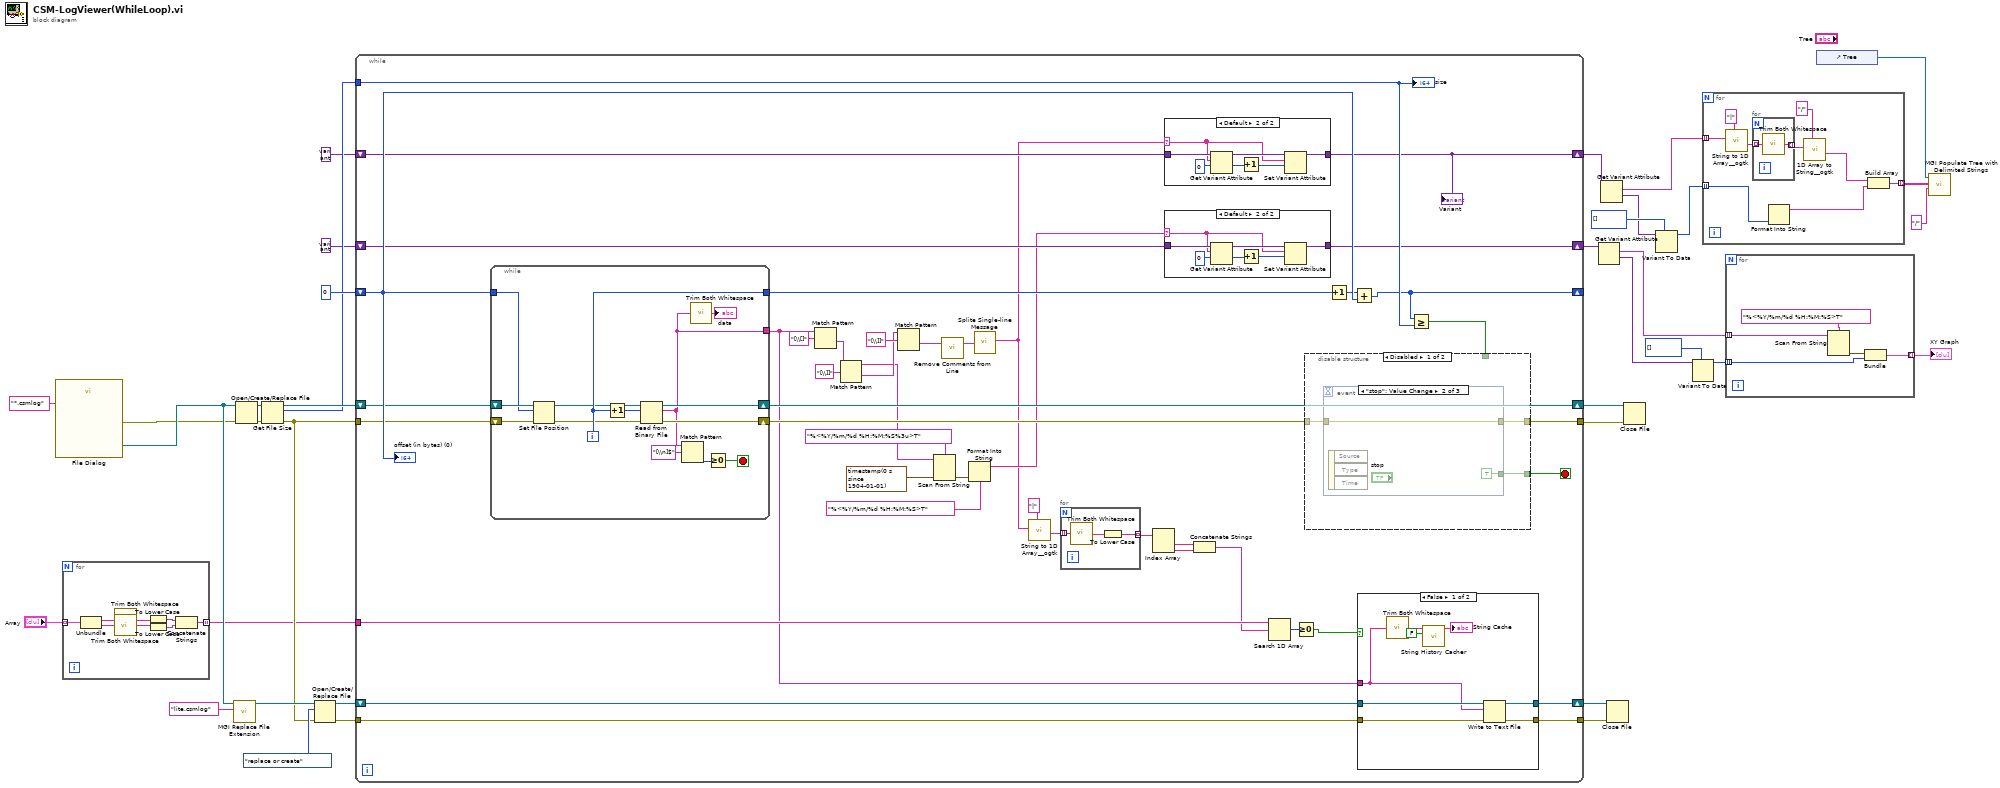
[diagram p0: block diagram]
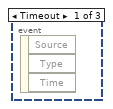
[diagram p5: hidden frame]
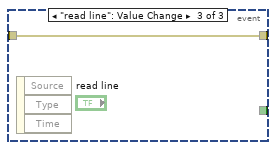
[diagram p6: hidden frame]
diagram:
  n1 = call "File Dialog"("pattern (all files)"="*.csmlog") -> ("selected path"=w11:path, "error out"=w8:errorcluster)  [unwired: 11 in, 2 out]
  n2 = for {
    tunnel: "Array" -> [w44] mode=indexing
    tunnel: [w41] -> w3 mode=indexing
    n3 = Unbundle(w44) -> ("CSM"=w43:string, "Message"=w42:string)
    n4 = call <userlib>:"Trim Both Whitespace.vi"("string"=w43) -> ("trimmed string"=w37:string)  [unwired: 1 in]
    n5 = call <userlib>:"Trim Both Whitespace.vi"("string"=w42) -> ("trimmed string"=w38:string)  [unwired: 1 in]
    n6 = To Lower Case(string=w37) -> (all lower case string=w40:string)
    n7 = To Lower Case(string=w38) -> (all lower case string=w39:string)
    n8 = Concatenate Strings(w40, w39) -> (w41:string)
  }
  n9 = call <userlib>:"MGI Replace File Extension.vi"("New Extension (txt)"="lite.csmlog", "Path In"=w11) -> ("Path Out"=w10:path)  [unwired: 8 in, 1 out]
  n10 = Open/Create/Replace File(file path (use dialog)=w11, error in=w8) -> (refnum out=w36:refnum<file>, error out=w35:errorcluster)  [unwired: 4 in, 1 out]
  n11 = Get File Size(file=w36, error in=w35) -> (refnum out=w33:refnum<file>, size (in bytes)=w30:i64, 0:w7:errorcluster)
  n12 = Open/Create/Replace File(file path (use dialog)=w10, error in=w7, operation (0:open)=T2."replace or create") -> (refnum out=w6:refnum<file>, error out=w5:errorcluster)  [unwired: 3 in, 1 out]
  n13 = while {
    shift-right: [w88] -> w31
    shift-left: w33 -> [w82]
    tunnel: [w85] -> w32
    shift-right: [w72] -> _
    shift-left: i64 0 ("offset (in bytes) (0)") -> [w83]
    tunnel: w7 -> [w81]
    tunnel: w30 -> [w79]
    shift-right: [w73] -> w23
    shift-left: variant -> [w74]
    shift-right: [w66] -> w19
    shift-left: variant -> [w67]
    tunnel: w5 -> [w54]
    shift-right: [w51] -> w1
    shift-left: w6 -> [w52]
    tunnel: w3 -> [w57]
    tunnel: [w53] -> w2
    stop <- w86 stop-if-true
    n14 = while {
      shift-right: [w130] -> w84
      shift-left: w81 -> [w124]
      shift-right: [w131] -> w88
      shift-left: w82 -> [w121]
      tunnel: [w125] -> w87
      tunnel: w83 -> [w120]
      tunnel: [w119] -> w45
      i -> [w125]
      stop <- w127 stop-if-true
      n15 = Set File Position(offset (in bytes) (0)=w120, refnum=w121, error in=w124) -> (refnum out=w122:refnum<file>, error out=w123:errorcluster)  [unwired: 1 in]
      n16 = Increment(x=w125) -> (x+1=w126:i32)
      n17 = Read from Binary File(8:w123, 10:w126, 11:w122) -> (0:w130:errorcluster, 2:w119:string, 3:w131:refnum<file>)  [unwired: 3 in, 1 out]
      n18 = Match Pattern(string=w119, regular expression="[\\n]$") -> (offset past match=w128:i32)  [unwired: 1 in, 3 out]
      n19 = call <userlib>:"Trim Both Whitespace.vi"("string"=w119) -> ("trimmed string"=→"data":string)  [unwired: 1 in]
      n20 = Greater Or Equal To 0?(x=w128) -> (x >= 0?=w127:bool)
    }
    n21 = Match Pattern(string=w45, regular expression="[\\[]") -> (after substring=w76:string)  [unwired: 1 in, 3 out]
    n22 = Match Pattern(string=w76, regular expression="[\\]]") -> (before substring=w65:string, after substring=w69:string)  [unwired: 1 in, 2 out]
    n23 = Match Pattern(string=w69, regular expression="[\\]]") -> (after substring=w68:string)  [unwired: 1 in, 3 out]
    n24 = Scan From String(format string="%<%Y/%m/%d %H:%M:%S%3u>T", input string=w65, default 1=timestamp(0 s since 1904-01-01)) -> (output 1=w62:timestamp)  [unwired: 2 in, 3 out]
    n25 = call <userlib>:"Remove Comments from Line.vi"("single-line text"=w68) -> ("single-line text without comments"=w71:string)  [unwired: 2 in]
    n26 = Format Into String(format string="%<%Y/%m/%d %H:%M:%S>T", w62) -> (resulting string=w60:string)  [unwired: 2 in, 1 out]
    n27 = call <userlib>:"Splite Single-line Message.vi"("single-line text"=w71) -> ("state"=w49:string)  [unwired: 6 in, 3 out]
    n28 = call <userlib>:"String to 1D Array__ogtk.vi"("delimiter (Tab)"="|", "string"=w49) -> ("Array of Strings"=w58:string[])  [unwired: 9 in]
    n29 = for {
      tunnel: w58 -> [w101] mode=indexing
      tunnel: [w99] -> w56 mode=indexing
      n30 = call <userlib>:"Trim Both Whitespace.vi"("string"=w101) -> ("trimmed string"=w100:string)  [unwired: 1 in]
      n31 = To Lower Case(string=w100) -> (all lower case string=w99:string)
    }
    n32 = Index Array(array=w56) -> (element #1=w48:string, element #2=w47:string)  [unwired: 2 in]
    n33 = case shown="Default" w49 {
      selector: w49 -> [_ w103]
      tunnel: w67 -> [w102 w109]
      tunnel: [w102 w105] -> w66
      frame "" {
      }
      frame Default {
        n34 = Get Variant Attribute(Variant=w109, name=w103, default value (empty Variant)=i64 0 ("offset (in bytes) (0)")) -> (duplicate Variant=w106:variant, value=w107:i64)  [unwired: 1 in, 2 out]
        n35 = Increment(x=w107) -> (x+1=w104:i64)
        n36 = Set Variant Attribute(Variant=w106, name=w103, value=w104) -> (Variant out=w105:variant)  [unwired: 1 in, 2 out]
      }
    }
    "Variant" <- w66
    n37 = case shown="Default" w60 {
      selector: w60 -> [_ w111]
      tunnel: w74 -> [w110 w117]
      tunnel: [w110 w113] -> w73
      frame "" {
      }
      frame Default {
        n38 = Get Variant Attribute(Variant=w117, name=w111, default value (empty Variant)=i64 0 ("offset (in bytes) (0)")) -> (duplicate Variant=w114:variant, value=w115:i64)  [unwired: 1 in, 2 out]
        n39 = Increment(x=w115) -> (x+1=w112:i64)
        n40 = Set Variant Attribute(Variant=w114, name=w111, value=w112) -> (Variant out=w113:variant)  [unwired: 1 in, 2 out]
      }
    }
    n41 = Concatenate Strings(w48, w47) -> (w46:string)
    n42 = Search 1D Array(1D array=w57, element=w46) -> (index of element=w55:i32)  [unwired: 1 in]
    n43 = Greater Or Equal To 0?(x=w55) -> (x >= 0?=w50:bool)
    n44 = Increment(x=w87) -> (x+1=w80:i32)
    n45 = Add(x=w80, y=w83) -> (x+y=w72:i64)
    n46 = case shown="False" w50 {
      tunnel: w54 -> [w96 w98]
      tunnel: [w95 w98] -> w53
      tunnel: w52 -> [w94 w97]
      tunnel: [w93 w97] -> w51
      tunnel: w45 -> [w91 _]
      frame False {
        n47 = call <userlib>:"Trim Both Whitespace.vi"("string"=w91) -> ("trimmed string"=w89:string)  [unwired: 1 in]
        n48 = call <userlib>:"String History Cacher.vi"("Include Timestamp(T)"=FALSE, "String"=w89) -> ("String Cache"=→"String Cache":string)  [unwired: 9 in]
        n49 = Write to Text File(file (use dialog)=w94, text=w91, error in=w96) -> (refnum out=w93:refnum<file>, error out=w95:errorcluster)  [unwired: 1 in, 1 out]
      }
      frame True {
      }
    }
    n50 = Greater Or Equal?(x=w72, y=w79) -> (x >= y?=w78:bool)
    n51 = disable-structure shown="Disabled" {
      disable-tunnel: [w134 w138] -> w86
      disable-tunnel: [w133 _] -> w85
      disable-tunnel: w84 -> [w132 _]
      disable-tunnel: w78 -> [_ w138]
      frame Disabled {
        n52 = event shown="[1] \"stop\": Value Change" {
          selector: _ -> [_ _ _]
          dyn-events: _ -> [_ _ _]
          timeout: _ -> [_ _ _]
          tunnel: [_ TRUE ("stop") _] -> w134
          tunnel: [_ w136 w137] -> w133
          tunnel: w132 -> [_ w136 w137]
          event Timeout {
            n53 = event-data() -> ()  [unwired: 1 in, 3 out]
          }
          event "stop": Value Change {
            n54 = event-data() -> ()  [unwired: 1 in, 3 out]
          }
          event "read line": Value Change {
            n55 = event-data() -> ()  [unwired: 1 in, 3 out]
          }
        }
      }
      frame Enabled {
      }
    }
    "offset (in bytes) (0)" <- w83
    "size" <- w79
  }
  n56 = Get Variant Attribute(Variant=w23) -> (names=w25:string[], values=w26:variant[])  [unwired: 3 in, 2 out]
  n57 = Get Variant Attribute(Variant=w19) -> (names=w18:string[], values=w20:variant[])  [unwired: 3 in, 2 out]
  n58 = Close File(refnum=w1, error in=w2) -> ()  [unwired: 2 out]
  n59 = Close File(refnum=w31, error in=w32) -> ()  [unwired: 2 out]
  n60 = Variant To Data(type=i64[] [] ("offset (in bytes) (0)"), Variant=w20) -> (data=w17:i64[])  [unwired: 1 in, 1 out]
  n61 = Variant To Data(type=i64[] [] ("offset (in bytes) (0)"), Variant=w26) -> (data=w27:i64[])  [unwired: 1 in, 1 out]
  n62 = for {
    tunnel: w18 -> [w147] mode=indexing
    tunnel: w17 -> [w141] mode=indexing
    tunnel: [w139] -> w16 mode=indexing
    n63 = call <userlib>:"String to 1D Array__ogtk.vi"("delimiter (Tab)"="|", "string"=w147) -> ("Array of Strings"=w145:string[])  [unwired: 9 in]
    n64 = for {
      tunnel: w145 -> [w149] mode=indexing
      tunnel: [w148] -> w144 mode=indexing
      n65 = call <userlib>:"Trim Both Whitespace.vi"("string"=w149) -> ("trimmed string"=w148:string)  [unwired: 1 in]
    }
    n66 = Format Into String(w141) -> (resulting string=w140:string)  [unwired: 3 in, 1 out]
    n67 = call <userlib>:"1D Array to String__ogtk.vi"("delimiter (Tab)"="/", "Array of Strings"=w144) -> ("delimited string"=w142:string)  [unwired: 9 in]
    n68 = Build Array(w142, w140) -> (w139:string[])
  }
  n69 = for {
    tunnel: w25 -> [w153] mode=indexing
    tunnel: w27 -> [w151] mode=indexing
    tunnel: [w150] -> w28 mode=indexing
    n70 = Scan From String(format string="%<%Y/%m/%d %H:%M:%S>T", input string=w153) -> (output 1=w152:timestamp)  [unwired: 3 in, 3 out]
    n71 = Bundle(w152, "offset (in bytes) (0)"=w151) -> (w150:cluster{timestamp, "offset (in bytes) (0)":i64})  [unwired: 1 in]
  }
  "XY Graph" <- w28
  n72 = control-ref of="Tree"() -> (w14:refnum<vi>)
  n73 = call <userlib>:"MGI Populate Tree with Delimited Strings.vi"("Delimiter"="/" ("delimiter (Tab)"), "Items (Delimited)"=w16, "Tree Control"=w14) -> ()  [unwired: 6 in, 3 out]
